vi "Debug Display.vi"() -> ()   [LabVIEW 2011]
panel:
  out "Wheel Pos/Speed":picture
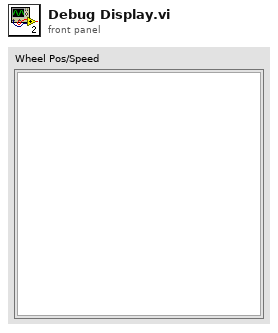
[diagram p1: front panel]
types:
  T1 = cluster{"Array of Int16[0]":i16, "Array of Int16[1]":i16, "Array of Int16[2]":i16, "Array of Int16[3]":i16, "Array of Int16[4]":i16, "Array of Int16[5]":i16, "Array of Int16[6]":i16, "Array of Int16[7]":i16, "Array of Int16[8]":i16}
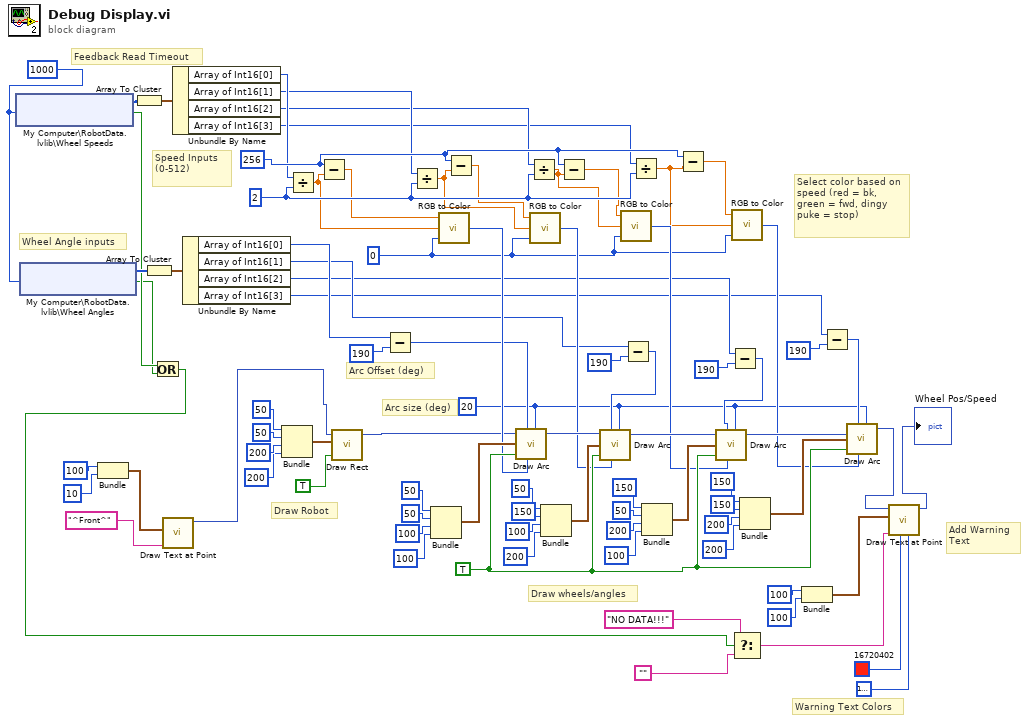
[diagram p0: block diagram]
diagram:
  w9 = 1000
  w32 = 20
  w34 = 0
  w50 = 2
  w51 = 256
  w63 = TRUE
  # "Add Warning\nText"
  # "Warning Text Colors"
  # "Feedback Read Timeout"
  # "Arc Offset (deg)"
  # "Arc size (deg)"
  # "Speed Inputs (0-512)"
  # "Wheel Angle inputs"
  # "Draw wheels/angles"
  # "Select color based on speed (red = bk, green = fwd, dingy puke = stop)"
  # "Draw Robot"
  n1 = shared-variable "My Computer\\RobotData.lvlib\\Wheel Speeds"(w9) -> (w26:i16[], w8:bool)  [unwired: 1 in, 1 out]
  n2 = shared-variable "My Computer\\RobotData.lvlib\\Wheel Angles"(w9) -> (w25:i16[], w7:bool)  [unwired: 1 in, 1 out]
  n3 = Bundle(100, 10) -> (w27:cluster{i32, i32})  [unwired: 1 in]
  n4 = Array To Cluster(array=w26) -> (cluster=w24:T1)
  n5 = Array To Cluster(array=w25) -> (cluster=w23:T1)
  n6 = Or(x=w8, y=w7) -> (x .or. y?=w6:bool)
  n7 = call <vilib>:"Draw Text at Point.vi"("text"="^Front^", "origin"=w27) -> ("new picture"=w31:picture)  [unwired: 8 in, 1 out]
  n8 = Unbundle By Name(w24) -> ("Array of Int16[0]"=w22:i16, "Array of Int16[1]"=w21:i16, "Array of Int16[2]"=w20:i16, "Array of Int16[3]"=w19:i16)
  n9 = Unbundle By Name(w23) -> ("Array of Int16[0]"=w18:i16, "Array of Int16[1]"=w17:i16, "Array of Int16[2]"=w16:i16, "Array of Int16[3]"=w15:i16)
  n10 = Bundle(50, 50, 200, 200) -> (w54:cluster{i32, i32, i32, i32})  [unwired: 1 in]
  n11 = Divide(x=w22, y=w50) -> (x/y=w49:dbl)
  n12 = Subtract(x=w51, y=w49) -> (x-y=w46:dbl)
  n13 = call <vilib>:"Draw Rect.vi"("picture"=w31, "rect"=w54, "fill?(F)"=TRUE) -> ("new picture"=w52:picture)  [unwired: 6 in]
  n14 = Subtract(x=w18, y=190) -> (x-y=w40:i32)
  n15 = Divide(x=w21, y=w50) -> (x/y=w48:dbl)
  n16 = Bundle(50, 50, 100, 100) -> (w80:cluster{i32, i32, i32, i32})  [unwired: 1 in]
  n17 = call <vilib>:"RGB to Color.vi"("B"=w34, "G"=w49, "R"=w46) -> ("Color"=w62:u32)
  n18 = Subtract(x=w51, y=w48) -> (x-y=w45:dbl)
  n19 = call <vilib>:"Draw Arc.vi"("picture"=w52, "start angle[degrees]"=w40, "rect"=w80, "fill?(F)"=w63, "color(black)"=w62, "arc size[degrees]"=w32) -> ("new picture"=w86:picture)  [unwired: 3 in]
  n20 = Divide(x=w20, y=w50) -> (x/y=w44:dbl)
  n21 = call <vilib>:"RGB to Color.vi"("B"=w34, "G"=w48, "R"=w45) -> ("Color"=w61:u32)
  n22 = Bundle(50, 150, 100, 200) -> (w66:cluster{i32, i32, i32, i32})  [unwired: 1 in]
  n23 = Subtract(x=w51, y=w44) -> (x-y=w43:dbl)
  n24 = call <vilib>:"RGB to Color.vi"("B"=w34, "G"=w44, "R"=w43) -> ("Color"=w60:u32)
  n25 = Subtract(x=w17, y=190) -> (x-y=w36:i32)
  n26 = call <vilib>:"Draw Arc.vi"("picture"=w86, "start angle[degrees]"=w36, "rect"=w66, "fill?(F)"=w63, "color(black)"=w61, "arc size[degrees]"=w32) -> ("new picture"=w85:picture)  [unwired: 3 in]
  n27 = Divide(x=w19, y=w50) -> (x/y=w47:dbl)
  n28 = Bundle(150, 50, 200, 100) -> (w65:cluster{i32, i32, i32, i32})  [unwired: 1 in]
  n29 = Subtract(x=w51, y=w47) -> (x-y=w42:dbl)
  n30 = Subtract(x=w16, y=190) -> (x-y=w35:i32)
  n31 = call <vilib>:"Draw Arc.vi"("picture"=w85, "start angle[degrees]"=w35, "rect"=w65, "fill?(F)"=w63, "color(black)"=w60, "arc size[degrees]"=w32) -> ("new picture"=w84:picture)  [unwired: 3 in]
  n32 = call <vilib>:"RGB to Color.vi"("B"=w34, "G"=w47, "R"=w42) -> ("Color"=w59:u32)
  n33 = Select(t="NO DATA!!!", s=w6, f="") -> (s? t:f=w3:string)
  n34 = Bundle(150, 150, 200, 200) -> (w64:cluster{i32, i32, i32, i32})  [unwired: 1 in]
  n35 = Bundle(100, 100) -> (w10:cluster{i32, i32})  [unwired: 1 in]
  n36 = Subtract(x=w15, y=190) -> (x-y=w33:i32)
  n37 = call <vilib>:"Draw Arc.vi"("picture"=w84, "start angle[degrees]"=w33, "rect"=w64, "fill?(F)"=w63, "color(black)"=w59, "arc size[degrees]"=w32) -> ("new picture"=w14:picture)  [unwired: 3 in]
  n38 = call <vilib>:"Draw Text at Point.vi"("BG color(transparent)"=u32 16777216, "text color(black)"=u32 16720402, "text"=w3, "origin"=w10, "picture"=w14) -> ("new picture"=→"Wheel Pos/Speed":picture)  [unwired: 5 in, 1 out]
